vi "cos_2fs.vi"() -> ()   [LabVIEW 2009]
uses:
  <vilib>/imath/engines/lvmath2/RunTimeEngine/ErrorHandling/NIMS_Finalize Error.vi
  <vilib>/imath/engines/lvmath2/RunTimeEngine/Parser/MC_Version.vi
  <vilib>/imath/engines/lvmath2/RunTimeEngine/Managers/WorkSpace/UID Generator.vi
  <vilib>/imath/engines/lvmath2/RunTimeEngine/NodeEndStatement/NIMS_NodeEndStatement_Output.vi
  <instcachedir>/0/NIMS_NodeEndStatement_Output_53EC0D466D134D7ABD903AC30B43404B.lvgen/NIMS_NodeEndStatement_Output_53EC0D466D134D7ABD903AC30B43404B_001.vi
  <vilib>/imath/engines/lvmath2/RunTimeEngine/Managers/SymbolTable/Clear UID.vi
  <vilib>/imath/engines/lvmath/Plug In/_Char/NIMS_CH_character datatype.ctl
  <vilib>/imath/engines/lvmath2/RunTimeEngine/LocalVariableDefStatement/MC_LocalVariableDefStatement_Display.vi
  <vilib>/imath/engines/lvmath/Functions/Error Handling/MergeErrorsWrapper.vi
  <vilib>/imathl/engines/lvmath/Functions/Error Handling/Create Error.vi
  <vilib>/imath/engines/lvmath/Functions/Error Handling/MC_Error Cluster From Error Code.vi
  <vilib>/imath/engines/lvmath2/RunTimeEngine/RunTimeType/NIMS_RunTimeType_From StrictType (excl LVString).vi
  <vilib>/imath/engines/lvmath/Plug In/_Char/NIMS_CH_String to Character Array.vi
  <vilib>/imath/engines/lvmath2/RunTimeEngine/BuiltInFunctions/num_to_str/NIMS_num_to_str(GRowV,I32).vi
  <instcachedir>/0/NIMS_num_to_str(GRowV,I32)_52FF5984ECAE430BAA47FE5E9FC630B0.lvgen/NIMS_num_to_str(GRowV,I32)_52FF5984ECAE430BAA47FE5E9FC630B0_000.vi
  <vilib>/imath/engines/lvmath2/RunTimeEngine/RangeToken/NIMS_Range.vi
  <instcachedir>/0/NIMS_Range_08574DECC23E450FAF0AC0BC39E6BEA7.lvgen/NIMS_Range_08574DECC23E450FAF0AC0BC39E6BEA7_000.vi
  <vilib>/imath/engines/lvmath2/RunTimeEngine/ArithmeticOperatorToken/NIMS_ArithmeticOperator_plus.vi
  <instcachedir>/0/NIMS_ArithmeticOperator_plus_48B9519178ED42D7840F01273E784BFE.lvgen/NIMS_ArithmeticOperator_plus_48B9519178ED42D7840F01273E784BFE_001.vi
  <vilib>/imath/engines/lvmath2/RunTimeEngine/BuiltInFunctions/fft/NIMS_fft(GV).vi
  <instcachedir>/0/NIMS_fft(GV)_4C6467FC22F84E4BA42517A07EF978B0.lvgen/NIMS_fft(GV)_4C6467FC22F84E4BA42517A07EF978B0_000.vi
  <vilib>/imath/engines/lvmath2/RunTimeEngine/BuiltInFunctions/abs/NIMS_abs(signed).vi
  <instcachedir>/0/NIMS_abs(signed)_C4FCB8E6058B49B797C7C8D53CA5F6EC.lvgen/NIMS_abs(signed)_C4FCB8E6058B49B797C7C8D53CA5F6EC_000.vi
  <vilib>/imath/engines/lvmath2/RunTimeEngine/VariableToken/Read/NIMS_Get Elements - RV(_) - Check.vi
  <instcachedir>/0/NIMS_Get Elements - RV(_) - Check_30A5434E2C4242B098C990FE3FB371BC.lvgen/NIMS_Get Elements - RV(_) - Check_30A5434E2C4242B098C990FE3FB371BC_001.vi
  <instcachedir>/0/NIMS_num_to_str(GRowV,I32)_52FF5984ECAE430BAA47FE5E9FC630B0.lvgen/NIMS_num_to_str(GRowV,I32)_52FF5984ECAE430BAA47FE5E9FC630B0_001.vi
  <instcachedir>/0/NIMS_Get Elements - RV(_) - Check_30A5434E2C4242B098C990FE3FB371BC.lvgen/NIMS_Get Elements - RV(_) - Check_30A5434E2C4242B098C990FE3FB371BC_002.vi
  <vilib>/imath/engines/lvmath2/RunTimeEngine/Managers/SymbolTable/NIMS_WorkSpace.lvlib
panel:
  out "Power dB":dbl[](graph)
  out "Power Watts":dbl[](graph)
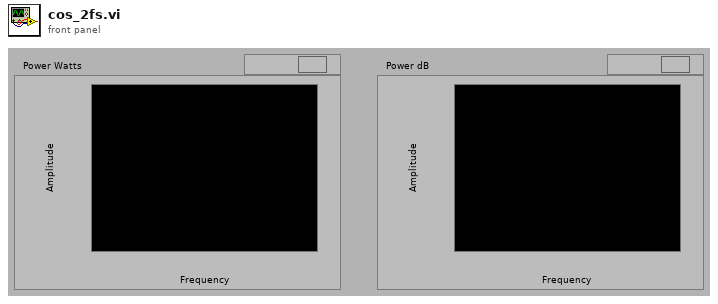
[diagram p1: front panel]
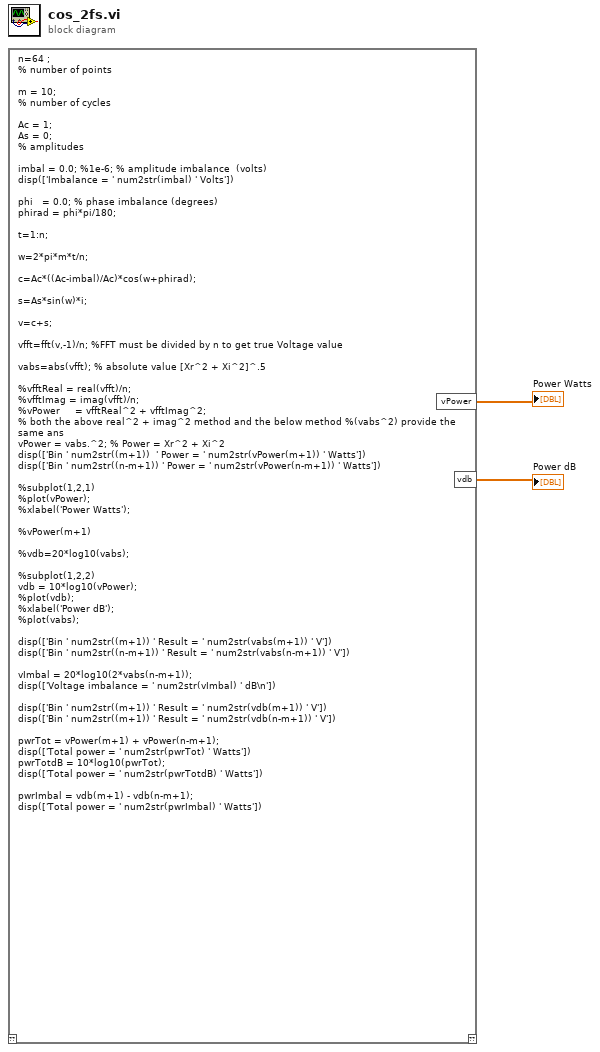
[diagram p0: block diagram]
diagram:
  n1 = mathscript code="n=64 ;\n% number of points\n\nm = 10;\n% number of cycles\n\nAc = 1;\nAs = 0;\n% amplitudes\n\nimbal = 0.0; %1e-6; % amplitude imbalance  (volts)\ndisp(['Imbalance = ' num2str(imbal) ' Volts'])\n\nphi   = 0.0; % phase imbalance (degrees)\nphirad = phi*pi/180;\n\nt=1:n;\n\nw=2*pi*m*t/n;\n\nc=Ac*((Ac-imbal)/Ac)*cos(w+phirad);\n\ns=As*sin(w)*i;\n\nv=c+s;\n\nvfft=fft(v,-1)/n; %FFT must be divided by n to get true Voltage value\n\nvabs=abs(vfft); % absolute value [Xr^2 + Xi^2]^.5\n\n%vfftReal = real(vfft)/n;\n%vfftImag = imag(vfft)/n;\n%vPower     = vfftReal^2 + vfftImag^2;\n% both the above real^2 + imag^2 method and the below method %(vabs^2) provide the same ans\nvPower = vabs.^2; % Power = Xr^2 + Xi^2\ndisp(['Bin ' num2str((m+1))  ' Power = ' num2str(vPower(m+1)) ' Watts'])\ndisp(['Bin ' num2str((n-m+1)) ' Power = ' num2str(vPower(n-m+1)) ' Watts'])\n\n%subplot(1,2,1)\n%plot(vPower);\n%xlabel('Power Watts');\n\n%vPower(m+1)\n\n%vdb=20*log10(vabs);\n\n%subplot(1,2,2)\nvdb = 10*log10(vPower);\n%plot(vdb);\n%xlabel('Power dB');\n%plot(vabs);\n\ndisp(['Bin ' num2str((m+1)) ' Result = ' num2str(vabs(m+1)) ' V'])\ndisp(['Bin ' num2str((n-m+1)) ' Result = ' num2str(vabs(n-m+1)) ' V'])\n\nvImbal = 20*log10(2*vabs(n-m+1));\ndisp(['Voltage imbalance = ' num2str(vImbal) ' dB\\n'])\n\ndisp(['Bin ' num2str((m+1)) ' Result = ' num2str(vdb(m+1)) ' V'])\ndisp(['Bin ' num2str((m+1)) ' Result = ' num2str(vdb(n-m+1)) ' V'])\n\npwrTot = vPower(m+1) + vPower(n-m+1);\ndisp(['Total power = ' num2str(pwrTot) ' Watts'])\npwrTotdB = 10*log10(pwrTot);\ndisp(['Total power = ' num2str(pwrTotdB) ' Watts'])\n\npwrImbal = vdb(m+1) - vdb(n-m+1);\ndisp(['Total power = ' num2str(pwrImbal) ' Watts'])"() -> ("vPower"=→"Power Watts":dbl[], "vdb"=→"Power dB":dbl[])  [unwired: 1 in, 1 out]
